vi "test MSS.vi"(11 "Test Case In":refnum<class "Test HSU MCU V2.lvclass">) -> (0 "error out":errorcluster, 3 "Test Case Out":refnum<class "Test HSU MCU V2.lvclass">)   [LabVIEW 2024, in "Test HSU MCU V2.lvclass"]
uses:
  Test HSU MCU V2.lvclass
  C:/Program Files/National Instruments/LabVIEW 2024/vi.lib/Astemes/LUnit/Test Case.lvclass
  MSS/MSS.lvclass
  Virtual Instruments/Scaling Strategy/Scaling Strategy.lvclass
  Virtual Instruments/Perform Action Strategy/Perform Action Strategy.lvclass
  Perform Action HSU MCU Strategy/Perform Action HSU MCU Strategy.lvclass
  Virtual Instruments/No Scaling/No Scaling.lvclass
  <vilib>/Astemes/LUnit/Test Case.lvclass/Test Case.ctl
  <vilib>/Astemes/LUnit/Append Pass Result.vi
  <vilib>/Astemes/LUnit/Append Fail Result.vi
  <vilib>/Astemes/LUnit/Run In UI.vi
  <vilib>/Utility/error.llb/Clear Errors.vi
  <vilib>/Astemes/LUnit/Test Case.lvclass
panel:
  out "Output":variant
  out "Task-Point Ident":string
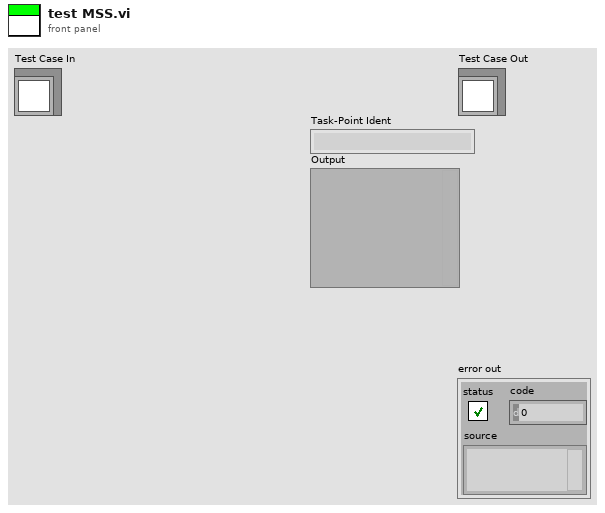
[diagram p1: front panel]
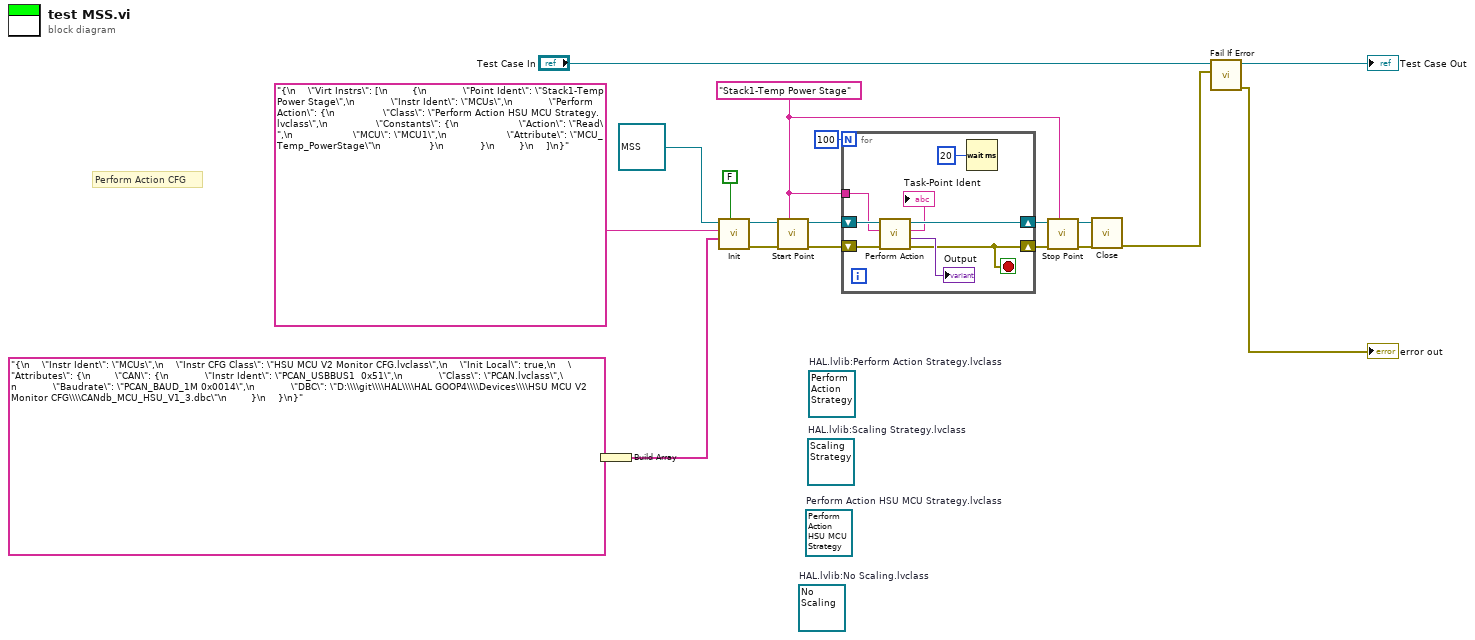
[diagram p0: block diagram]
diagram:
  (unwired) refnum<class "No Scaling.lvclass"> refnum  # HAL.lvlib:No Scaling.lvclass
  (unwired) refnum<class "Perform Action HSU MCU Strategy.lvclass"> refnum  # Perform Action HSU MCU Strategy.lvclass
  (unwired) refnum<class "Perform Action Strategy.lvclass"> refnum  # HAL.lvlib:Perform Action Strategy.lvclass
  (unwired) refnum<class "Scaling Strategy.lvclass"> refnum  # HAL.lvlib:Scaling Strategy.lvclass
  w1 = "Stack1-Temp Power Stage"
  # "Perform Action CFG"
  n1 = Build Array("{\n    \"Instr Ident\": \"MCUs\",\n    \"Instr CFG Class\": \"HSU MCU V2 Monitor CFG.lvclass\",\n    \"Init Local\": true,\n    \"Attributes\": {\n        \"CAN\": {\n            \"Instr Ident\": \"PCAN_USBBUS1  0x51\",\n            \"Class\": \"PCAN.lvclass\",\n            \"Baudrate\": \"PCAN_BAUD_1M 0x0014\",\n            \"DBC\": \"D:\\\\git\\\\HAL\\\\HAL GOOP4\\\\Devices\\\\HSU MCU V2 Monitor CFG\\\\CANdb_MCU_HSU_V1_3.dbc\"\n        }\n    }\n}") -> (w12:string[])
  n2 = call "Init.vi"("Is Target?"=FALSE, "Instr CFGs"=w12, "<JSON> Virt Instr CFG"="{\n    \"Virt Instrs\": [\n        {\n            \"Point Ident\": \"Stack1-Temp Power Stage\",\n            \"Instr Ident\": \"MCUs\",\n            \"Perform Action\": {\n                \"Class\": \"Perform Action HSU MCU Strategy.lvclass\",\n                \"Constants\": {\n                    \"Action\": \"Read\",\n                    \"MCU\": \"MCU1\",\n                    \"Attribute\": \"MCU_Temp_PowerStage\"\n                }\n            }\n        }\n    ]\n}", "MSS in"=refnum<class "MSS.lvclass"> refnum ("HAL.lvlib:MSS.lvclass")) -> ("error out"=w11:errorcluster, "MSS out"=w9:refnum<class "MSS.lvclass">)  [unwired: 4 in, 2 out]
  n3 = call "Start Point.vi"("Task-Point Ident"=w1, "error in"=w11, "MSS in"=w9) -> ("error out"=w10:errorcluster, "MSS out"=w5:refnum<class "MSS.lvclass">)  [unwired: 7 in]
  n4 = for {
    N: 100 -> [_]
    shift-right: [w20] -> w6
    shift-left: w10 -> [w27]
    shift-right: [w25] -> w4
    shift-left: w5 -> [w26]
    tunnel: w1 -> [w23]
    stop <- w20 stop-if-true
    n5 = call "Perform Action.vi"("error in"=w27, "Point Ident"=w23, "MSS in"=w26) -> ("error out"=w20:errorcluster, "Output"=→"Output":variant, "Task-Point Ident"=→"Task-Point Ident":string, "MSS out"=w25:refnum<class "MSS.lvclass">)  [unwired: 5 in]
    n6 = Wait (ms)(milliseconds to wait=u32 20) -> ()  [unwired: 1 out]
  }
  n7 = call "Stop Point.vi"("Task-Point Ident"=w1, "error in"=w6, "MSS in"=w4) -> ("error out"=w8:errorcluster, "MSS out"=w7:refnum<class "MSS.lvclass">)  [unwired: 7 in]
  n8 = call "Close.vi"("error in"=w8, "MSS in"=w7) -> ("error out"=w3:errorcluster)  [unwired: 8 in, 1 out]
  n9 = call <vilib>:"Fail If Error.vi"("Assert error"=w3, "LUnit Test Case In"="Test Case In") -> ("error out"=→"error out":errorcluster, "LUnit Test Case Out"=→"Test Case Out":refnum<class "Test HSU MCU V2.lvclass">)  [unwired: 8 in]
